vi "Event_Callback.vi"(4 "Variant":variant, 5 "Event Data":cluster{"deviceKey":string, "state":i32}, 6 "Control Ref":refnum<k24>, 7 "Event Common Data":T1) -> ()   [LabVIEW 2009]
uses:
  C:/Samples/LabVIEW/UseEventHandling/LabVIEW 2009/UsbDllWrap.dll
panel:
  in  "DeviceStateChangedEvent":refnum<user-event>
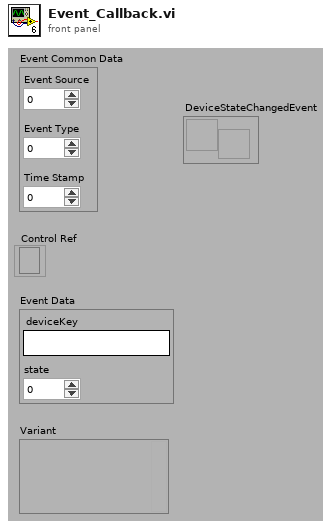
[diagram p1: front panel]
types:
  T1 = cluster{"Event Source":i32, "Event Type":u32, "Time Stamp":u32}
  T2 = cluster{"deviceKey":string, "new reference":refnum<k24>}
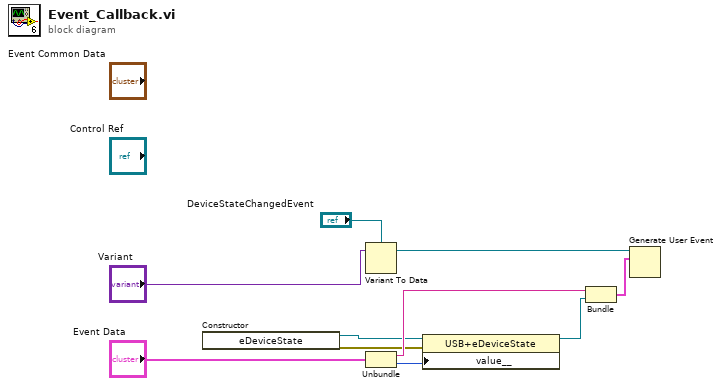
[diagram p0: block diagram]
diagram:
  n1 = constructor class="USB+eDeviceState"() -> (reference out=w2:refnum<k24>, error out=w1:errorcluster)  [unwired: 3 in, 1 out]
  n2 = Variant To Data(Variant="Variant", type="DeviceStateChangedEvent") -> (data=w9:refnum<user-event>)  [unwired: 1 in, 1 out]
  n3 = Unbundle("Event Data") -> ("deviceKey"=w5:string, "state"=w6:i32)
  n4 = property class="USB+eDeviceState"(reference=w2, error in=w1, "value__"=w6) -> (reference out=w4:refnum<k24>)  [unwired: 1 out]
  n5 = Bundle("deviceKey"=w5, "new reference"=w4) -> (w3:T2)  [unwired: 1 in]
  n6 = Generate User Event(user event=w9, event data cluster=w3) -> ()  [unwired: 1 in, 2 out]
